vi "LOAD USER PHOTO.vi"(10 "BYU ID #":string, 11 "connection reference in":T1) -> (2 "User Image":T2, 3 "connection reference out":T1)   [LabVIEW 2019]
uses:
  <vilib>/vision/Image Controls.llb/IMAQ Image.ctl
  <vilib>/addons/database/Connection.llb/Conn ObjectReference.ctl
  <vilib>/addons/database/NI_Database_API.lvlib
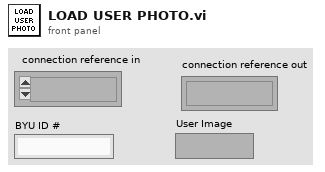
[diagram p1: front panel]
types:
  T1 = typedef "NI_Database_API.lvlib/Conn ObjectReference.ctl" = refnum<k1>
  T2 = typedef "IMAQ Image.ctl" = refnum<image>
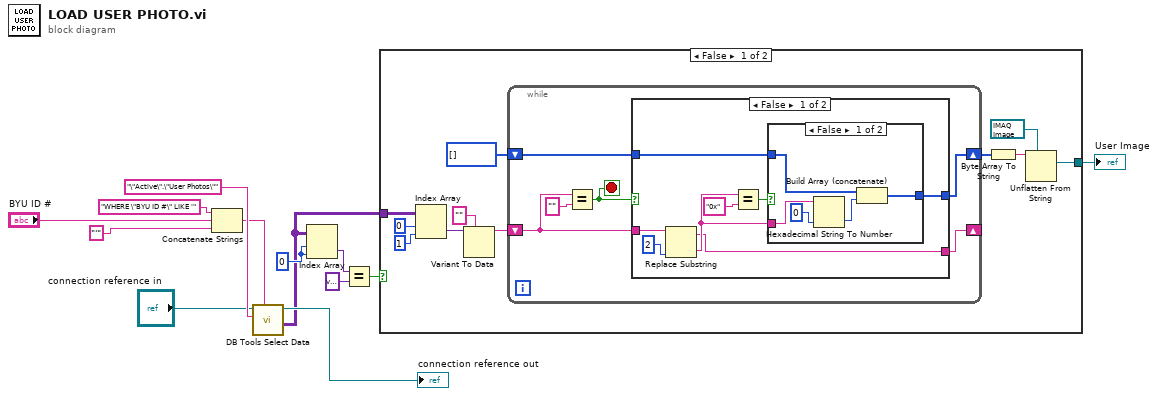
[diagram p0: block diagram]
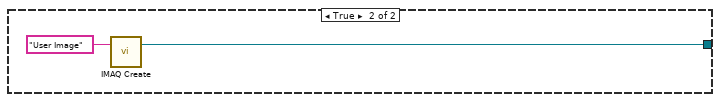
[diagram p4: hidden frame]
diagram:
  w13 = 0 ("disabled index (col)")
  n1 = Concatenate Strings("WHERE \"BYU ID #\" LIKE '", "BYU ID #", "'") -> (w3:string)
  n2 = call <vilib>:"DB Tools Select Data.vi"("condition"=w3, "table"="\"Active\".\"User Photos\"", "connection reference"="connection reference in") -> ("data"=w9:variant[][], "connection reference out"=→"connection reference out":T1)  [unwired: 3 in, 1 out]
  n3 = Index Array(array=w9, index (row)=w13, index (col)=w13) -> (element=w2:variant)
  n4 = Equal?(x=w2, y=variant) -> (x = y?=w10:bool)
  n5 = case shown="False" w10 {
    tunnel: w9 -> [w24 _]
    tunnel: [w14 w47] -> w8
    frame False {
      n6 = Index Array(array=w24, index (row)=0, index (col)=1 ("disabled index (col)")) -> (element=w20:variant)
      n7 = Variant To Data(type="" ("concatenated string"), Variant=w20) -> (data=w17:string)  [unwired: 1 in, 1 out]
      n8 = while {
        shift-right: [w25] -> _
        shift-left: w17 -> [w28]
        shift-right: [w29] -> w19
        shift-left: u8[] [] ("unsigned byte array") -> [w30]
        stop <- w26 stop-if-true
        n9 = Equal?(x=w28, y="") -> (x = y?=w26:bool)
        n10 = case shown="False" w26 {
          tunnel: w30 -> [w35 w45]
          tunnel: [w34 w45] -> w29
          tunnel: [w31 w46] -> w25
          tunnel: w28 -> [w32 w46]
          frame False {
            n11 = Replace Substring(2:2 ("length (len. of substring)"), 5:w32) -> (0:w33:string, 1:w31:string)  [unwired: 2 in]
            n12 = Equal?(x=w33, y="0x") -> (x = y?=w36:bool)
            n13 = case shown="False" w36 {
              tunnel: w35 -> [w41 w44]
              tunnel: [w39 w44] -> w34
              tunnel: w33 -> [w43 _]
              frame False {
                n14 = Hexadecimal String To Number(string=w43, default (0uL)=u8 0) -> (number=w40:u8)  [unwired: 1 in, 1 out]
                n15 = Build Array (concatenate)(w41, w40) -> (w39:u8[])
              }
              frame True {
              }
            }
          }
          frame True {
          }
        }
      }
      n16 = Byte Array To String(unsigned byte array=w19) -> (string=w15:string)
      n17 = Unflatten From String(type=T2 refnum ("New Image"), binary string=w15) -> (value=w14:T2)  [unwired: 3 in, 2 out]
    }
    frame True {
      n18 = call "IMAQ Create"("Image Name"="User Image") -> ("New Image"=w47:T2)  [unwired: 4 in, 1 out]
    }
  }
  "User Image" <- w8
